vi "JSONtext All Tests.vi"   [LabVIEW 2017]
uses:
  <vilib>/addons/_JKI Toolkits/Caraya/classes/Test/Test.lvclass
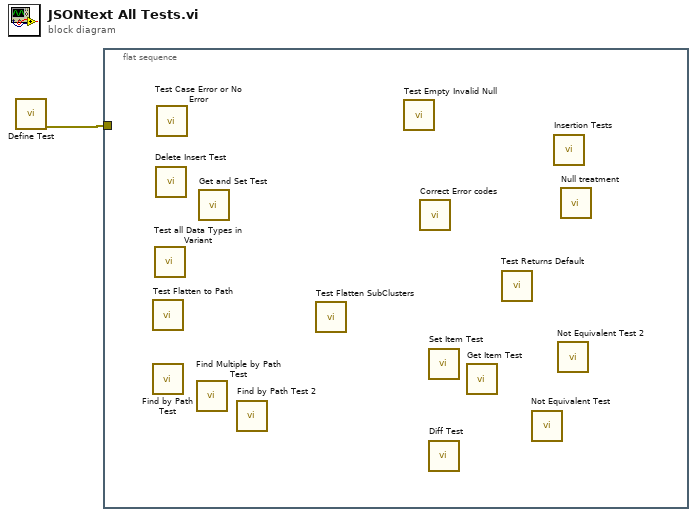
[diagram p0: block diagram]
diagram:
  n1 = call <vilib>:"Define Test.vi"() -> ("error out"=w1:errorcluster)  [unwired: 11 in]
  n2 = flat-sequence {
    tunnel: w1 -> [_]
    frame #0 {
      n3 = call "Test Flatten to Path.vi"() -> ()  [unwired: 12 in]
      n4 = call "Find by Path Test.vi"() -> ()  [unwired: 12 in]
      n5 = call "Test all Data Types in Variant.vi"() -> ()  [unwired: 12 in]
      n6 = call "Delete Insert Test.vi"() -> ()  [unwired: 12 in]
      n7 = call "Test Case Error or No Error.vi"() -> ()  [unwired: 12 in]
      n8 = call "Find Multiple by Path Test.vi"() -> ()  [unwired: 12 in]
      n9 = call "Get and Set Test.vi"() -> ()  [unwired: 12 in]
      n10 = call "Find by Path Test 2.vi"() -> ()  [unwired: 12 in]
      n11 = call "Test Flatten SubClusters.vi"() -> ()  [unwired: 12 in]
      n12 = call "Test Empty Invalid Null.vi"() -> ()  [unwired: 12 in]
      n13 = call "Correct Error codes.vi"() -> ()  [unwired: 12 in]
      n14 = call "Set Item Test.vi"() -> ()  [unwired: 12 in]
      n15 = call "Diff Test.vi"() -> ()  [unwired: 12 in]
      n16 = call "Get Item Test.vi"() -> ()  [unwired: 12 in]
      n17 = call "Test Returns Default.vi"() -> ()  [unwired: 12 in]
      n18 = call "Not Equivalent Test.vi"() -> ()  [unwired: 12 in]
      n19 = call "Insertion Tests.vi"() -> ()  [unwired: 12 in]
      n20 = call "Not Equivalent Test 2.vi"() -> ()  [unwired: 12 in]
      n21 = call "Null treatment.vi"() -> ()  [unwired: 12 in]
    }
  }
